vi "Solve2.vi"(8 "Error In":errorcluster, 11 "object in":refnum<class "2022_7.lvclass">) -> (0 "Error Out":errorcluster, 2 "Result":u64, 3 "object out":refnum<class "2022_7.lvclass">)   [LabVIEW 2020, in "2022_7.lvclass"]
uses:
  2022_7.lvclass
  2022_7.lvclass/2022_7.ctl
panel:
  out "Space Needed":i64
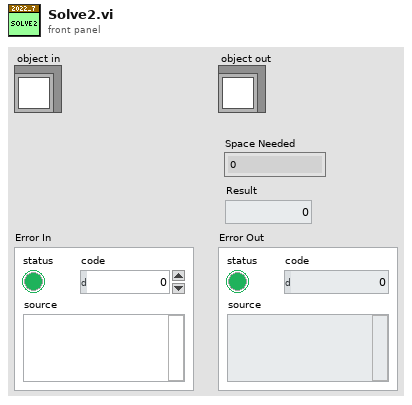
[diagram p1: front panel]
types:
  T1 = map{string[], cluster{"Folders":string[], "Files":cluster{"Name":string, "Size":i32}[]}}
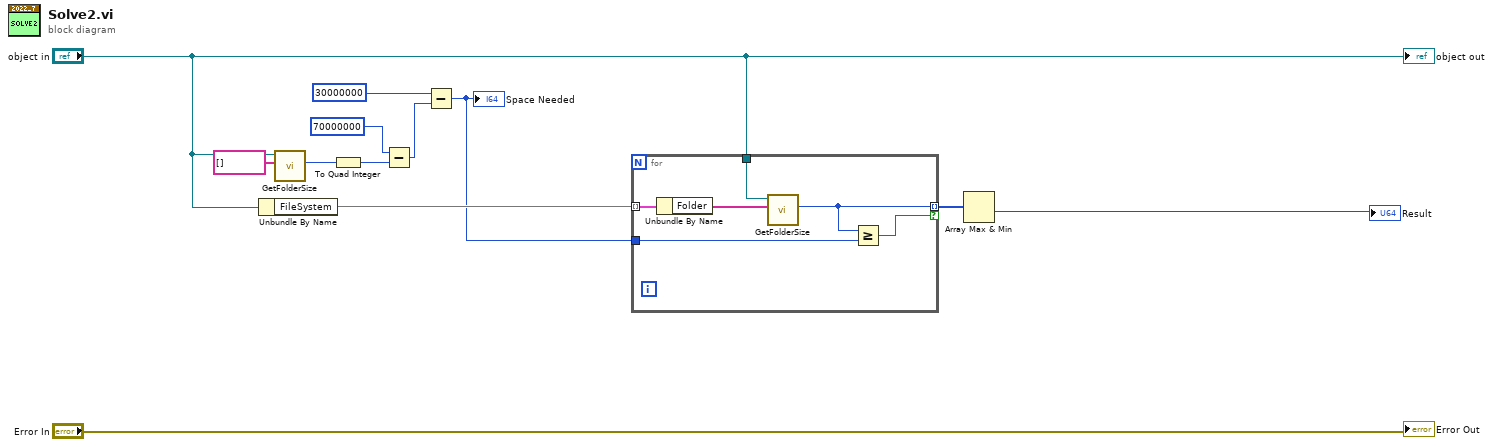
[diagram p0: block diagram]
diagram:
  n1 = Unbundle By Name("object in") -> ("FileSystem"=w11:T1)
  n2 = call "GetFolderSize.vi"("Folder"=string[] [], "object in"="object in") -> ("Size"=w7:u64)  [unwired: 7 in, 2 out]
  n3 = To Quad Integer(1:w7) -> (0:w4:i64)
  n4 = Subtract(x=i64 70000000, y=w4) -> (x-y=w6:i64)
  n5 = Subtract(x=i64 30000000, y=w6) -> (x-y=w3:i64)
  "Space Needed" <- w3
  n6 = for {
    tunnel: w11 -> [w18] mode=indexing
    tunnel: "object in" -> [w16]
    tunnel: [w15] -> w1 mode=indexing if=w14
    tunnel: w3 -> [w13]
    n7 = Unbundle By Name(w18) -> ("Folder"=w17:string[])
    n8 = call "GetFolderSize.vi"("Folder"=w17, "object in"=w16) -> ("Size"=w15:u64)  [unwired: 7 in, 2 out]
    n9 = Greater Or Equal?(x=w15, y=w13) -> (x >= y?=w14:bool)
  }
  n10 = Array Max & Min(array=w1) -> (min value=→"Result":u64)  [unwired: 3 out]
  "Error Out" <- "Error In"
  "object out" <- "object in"
